vi "Find Common Path.vi"(11 "Paths":path[](array[path])) -> (3 "Common Path":path)   [LabVIEW 2023]
doc: "Finds the common path between <B>Paths</B>."
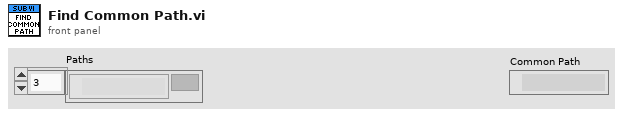
[diagram p1: front panel]
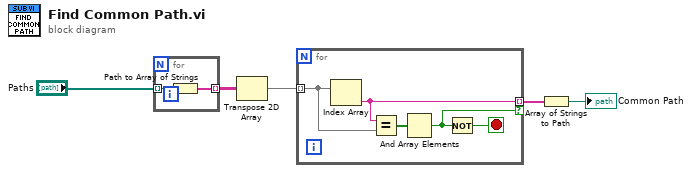
[diagram p0: block diagram]
diagram:
  n1 = for {
    tunnel: "Paths" -> [w7] mode=indexing
    tunnel: [w6] -> w2 mode=indexing
    n2 = Path to Array of Strings(0:w7) -> (2:w6:string[])  [unwired: 1 out]
  }
  n3 = Transpose 2D Array(2D array=w2) -> (transposed array=w4:string[][])
  n4 = for {
    tunnel: w4 -> [w10] mode=indexing
    tunnel: [w9] -> w1 mode=indexing if=w8
    stop <- w11 stop-if-true
    n5 = Index Array(array=w10) -> (element=w9:string)  [unwired: 1 in]
    n6 = Equal?(x=w9, y=w10) -> (x = y?=w12:bool[])
    n7 = And Array Elements(Boolean array=w12) -> (logical AND=w8:bool)
    n8 = Not(x=w8) -> (.not. x?=w11:bool)
  }
  n9 = Array of Strings to Path(0:w1) -> (2:→"Common Path":path)  [unwired: 1 in]
